vi "Get Category.vi"(8 "error in (no error)":errorcluster, 11 "dds editor node in":refnum<class "dds editor node.lvclass">) -> (0 "error out":errorcluster, 2 "Category":string, 3 "dds editor node out":refnum<class "dds editor node.lvclass">)   [LabVIEW 2020, in "dds editor node.lvclass"]
uses:
  dds editor node.lvclass
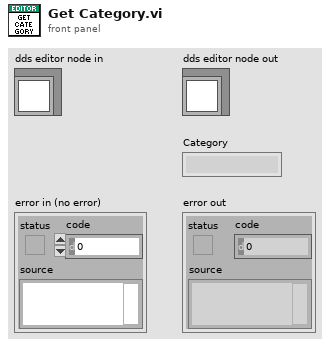
[diagram p1: front panel]
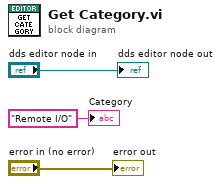
[diagram p0: block diagram]
diagram:
  "error out" <- "error in (no error)"
  "dds editor node out" <- "dds editor node in"
  "Category" <- "Remote I/O" ("Category")
